vi "displayHeartbeat.vi"() -> ()   [LabVIEW 2016, in "EXAViewElements.lvlib"]
doc: "Displays summary state information."
uses:
  EXAViewElements.lvlib
  ViewThisComponent/ViewThisComponent.lvclass
  home/andres/ct_cmpuserevents/ComponentTemplateCore/ComponentModel/ComponentModel/View/View.lvclass
  ComponentTemplateCore/ComponentModel/ComponentModel/View/View.lvclass
panel:
  in  "viewThisComponent":refnum<class "ViewThisComponent.lvclass">
  out "Heartbeat":bool
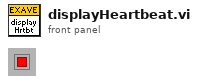
[diagram p1: front panel]
types:
  T1 = typedef "EXATypedefs.lvlib/PubDataEvents.ctl" = cluster{"DetailedState":refnum<user-event>, "ErrorCode":refnum<user-event>, "Heartbeat":refnum<user-event>, "LoopTime_ms":refnum<user-event>, "LoopTimeOutOfRange":refnum<user-event>, "RejectedCommand":refnum<user-event>, "SummaryState":refnum<user-event>, "Timestamp":refnum<user-event>}
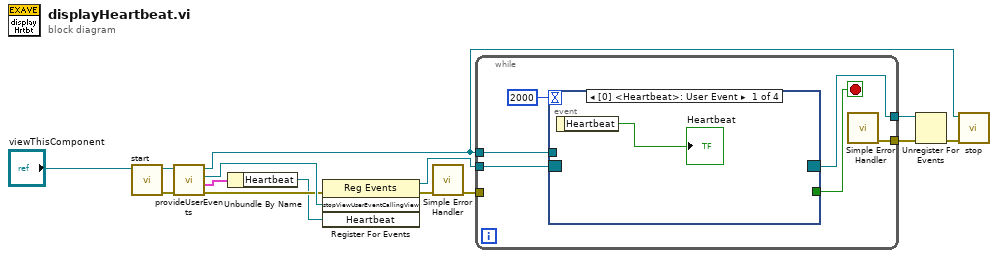
[diagram p0: block diagram]
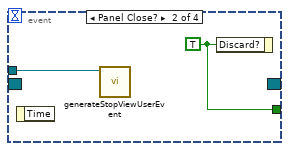
[diagram p2: hidden frame]
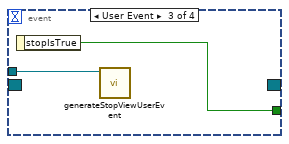
[diagram p3: hidden frame]
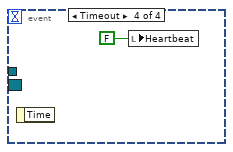
[diagram p4: hidden frame]
diagram:
  n1 = call-dynamic "start.vi"("View in"="viewThisComponent") -> ("error out"=w9:errorcluster, "View out"=w10:refnum<class "ViewThisComponent.lvclass">)  [unwired: 9 in]
  n2 = call "provideUserEvents.vi"("error in (no error)"=w9, "ViewThisComponent in"=w10) -> ("error out"=w11:errorcluster, "pubDataEvents"=w12:T1, "stopViewUserEventCallingView"=w13:refnum<user-event>, "ViewThisComponent out"=w5:refnum<class "ViewThisComponent.lvclass">)  [unwired: 6 in]
  n3 = Unbundle By Name(w12) -> ("Heartbeat"=w7:refnum<user-event>)
  n4 = register-events(error in=w11, w13, w7) -> (reference out=w6:refnum<event-registration>, error out=w14:errorcluster)  [unwired: 1 in]
  n5 = call <vilib>:"Simple Error Handler.vi"("error in (no error)"=w14) -> ("error out"=w4:errorcluster)  [unwired: 4 in, 4 out]
  n6 = while {
    tunnel: [w20] -> w3
    tunnel: w5 -> [w19]
    tunnel: w6 -> [w17]
    tunnel: w4 -> [_]
    tunnel: [w15] -> w1
    stop <- w16 stop-if-true
    n7 = event shown="[0] <Heartbeat>: User Event" {
      selector: w17 -> [_ _ _ _]
      dyn-events: [_ _ _ _] -> w15
      timeout: 2000 -> [_ _ _ _]
      tunnel: w19 -> [_ w23 w24 _]
      tunnel: [_ w22 w25 _] -> w16
      event User Event {
        n8 = event-data() -> ("Heartbeat"=→"Heartbeat":bool)  [unwired: 1 in]
      }
      event Panel Close? {
        w22 = TRUE
        n9 = event-data() -> ()  [unwired: 1 in, 1 out]
        n10 = call "generateStopViewUserEvent.vi"("View in"=w23) -> ()  [unwired: 9 in, 2 out]
        n11 = event-data("Discard?"=w22) -> ()  [unwired: 1 in, 1 out]
      }
      event User Event {
        n12 = event-data() -> ("stopIsTrue"=w25:bool)  [unwired: 1 in]
        n13 = call "generateStopViewUserEvent.vi"("View in"=w24) -> ()  [unwired: 9 in, 2 out]
      }
      event Timeout {
        n14 = event-data() -> ()  [unwired: 1 in, 1 out]
        n15 = local write "Heartbeat"(FALSE ("Heartbeat")) -> ()
      }
    }
    n16 = call <vilib>:"Simple Error Handler.vi"() -> ("error out"=w20:errorcluster)  [unwired: 5 in, 4 out]
  }
  n17 = Unregister For Events(event registration refnum=w1, error in=w3) -> (error out=w2:errorcluster)
  n18 = call-dynamic "stop.vi"("error in (no error)"=w2, "View in"=w5) -> ()  [unwired: 8 in, 2 out]
